vi "Show Error Details.vi"(8 "error in (no error)":errorcluster, 10 "Error Info":T1 {"Time Stamp" format="%<%x %.3X>T"}, 11 "Error Manager in":refnum<class "Local Error Manager.lvclass">) -> (0 "error out":errorcluster, 3 "Error Manager out":refnum<class "Local Error Manager.lvclass">)   [LabVIEW 2026, in "TALOS.lvlib" / "Error Manager.lvlib" / "Local Error Manager.lvclass"]
uses:
  Local Error Manager.lvclass
  C:/LabVIEW Code/TALOS/talos/Father of all uServices/Father of all uServices/Father of all uServices.lvclass
  Error Info.ctl
  Local Error Manager.lvclass/Local Error Manager.ctl
  Ancestor/Ancestor/Ancestor.lvclass/Ancestor.ctl
  <vilib>/AdvancedString/Delimited String to 1D String Array (string).vi
  Support VIs/Generate Error.vi
  FGV/Error Memory/Get Error Description.vi
  Support VIs/Get PC name.vi
  Ancestor/Ancestor/Read ID.vi
  Support VIs/Get Class Name.vi
  FGV/Error Memory/Error Memory Core.vi
  Support VIs/Circus Root Path.vi
  FGV/Error Memory/Error Crt Lvl checker.vi
  FGV/Error Memory/Error Memory Core.vi/40c8088d-b597-4017-91af-faa98e00292e.vi
  FGV/Error Memory/Error Memory Core.vi/d4a3ab98-063c-4e44-b43d-fbdcfe6c2be2.vi
  Support VIs/Global Memory.vi
  <vilib>/Utility/LVClass/Get LV Class Name.vi
  Support VIs/Is in Packed Library.vi
  Support VIs/TALOS Root path.vi
  Support VIs/Read CSV worksheet.vi
  Support VIs/Global Constants.vi
  <vilib>/Utility/error.llb/General Error Handler.vi
  Support VIs/Error Log.vi
  Ancestor/Ancestor/Ancestor.lvclass
  <vilib>/Comparison/Equal/Equal Functor/Equal Functor.lvclass
  Father of all uServices/Father of all uServices/Father of all uServices.lvclass
  TALOS.lvlib
  Error Manager.lvclass
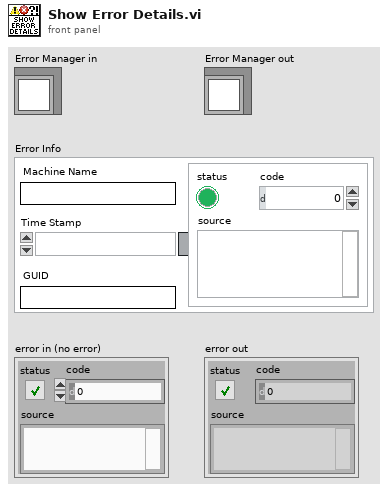
[diagram p1: front panel]
types:
  T1 = typedef "TALOS.lvlib/Error Manager.lvlib/Error Manager.lvclass/Error Info.ctl" = cluster{"error out":errorcluster, "Time Stamp":timestamp, "Machine Name":string, "GUID":string}
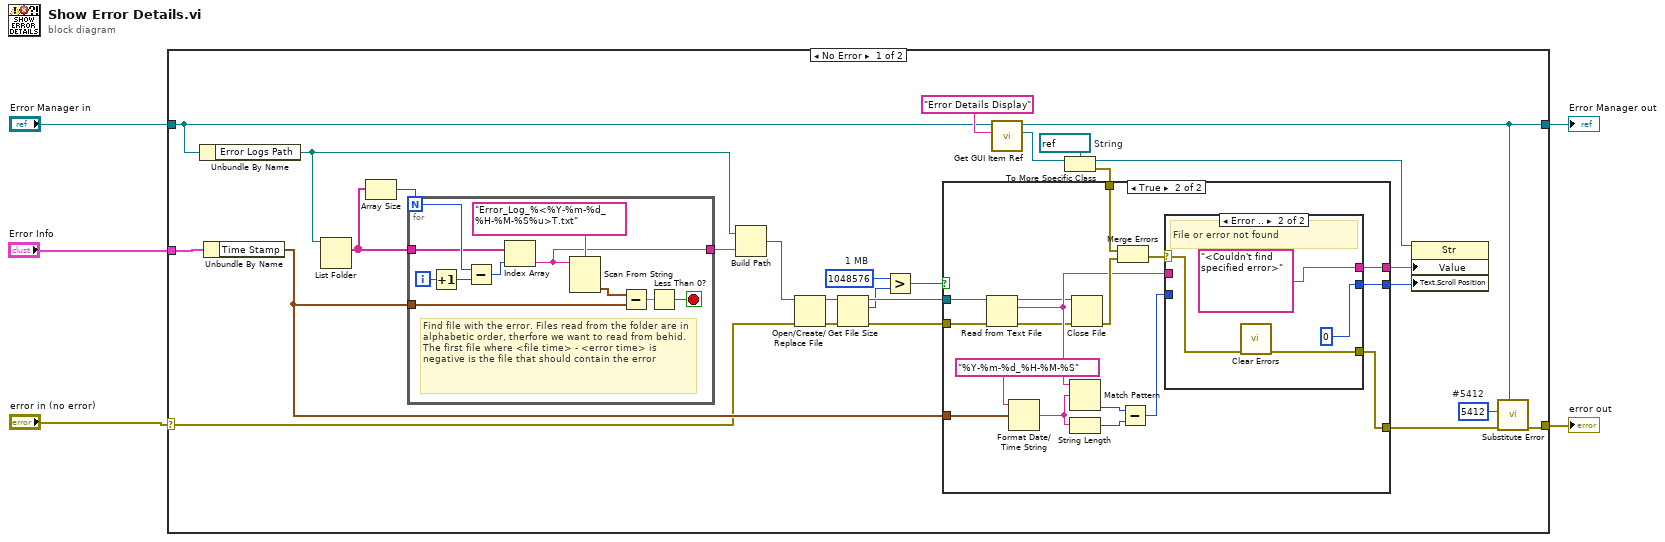
[diagram p0: block diagram]
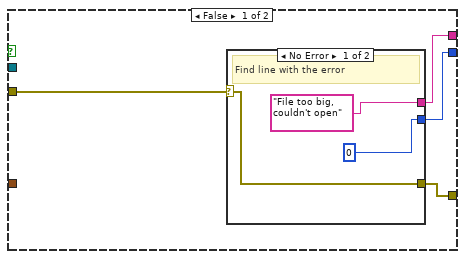
[diagram p2: hidden frame]
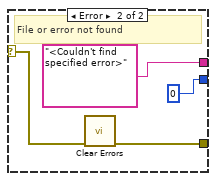
[diagram p3: hidden frame]
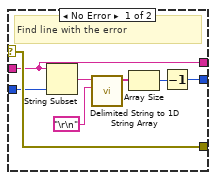
[diagram p4: hidden frame]
diagram:
  n1 = case shown="No Error" "error in (no error)" {
    selector: "error in (no error)" -> [w25 w84]
    tunnel: [w7 w84] -> w5
    tunnel: [w6 w85] -> w4
    tunnel: "Error Manager in" -> [w23 w85]
    tunnel: "Error Info" -> [w17 _]
    frame No Error {
      w9 = 5412  # #5412
      w11 = i64 1048576  # 1 MB
      w28 = refnum<vi> refnum  # String
      n2 = Unbundle By Name(w23) -> ("Error Logs Path"=w18:path)
      n3 = Unbundle By Name(w17) -> ("Time Stamp"=w29:timestamp)
      n4 = List Folder(path=w18) -> (filenames=w20:string[])  [unwired: 3 in, 3 out]
      n5 = Array Size(array=w20) -> (size(s)=w19:i32)
      n6 = for {
        N: w19 -> [w82]
        tunnel: w20 -> [w80]
        tunnel: w29 -> [w76]
        tunnel: [w73] -> w21
        i -> [w83]
        stop <- w74 stop-if-true
        # "Find file with the error. Files read from the folder are in alphabetic order, therfore we want to read from behid. The first file where <file time> - <error time> is negative is the file that should contain the error"
        n7 = Increment(x=w83) -> (x+1=w81:i32)
        n8 = Subtract(x=w82, y=w81) -> (x-y=w79:i32)
        n9 = Index Array(array=w80, index=w79) -> (element=w73:string)
        n10 = Scan From String(format string="Error_Log_%<%Y-%m-%d_%H-%M-%S%u>T.txt", input string=w73) -> (output 1=w77:timestamp)  [unwired: 3 in, 3 out]
        n11 = Subtract(x=w77, y=w76) -> (x-y=w75:dbl)
        n12 = Less Than 0?(x=w75) -> (x < 0?=w74:bool)
      }
      n13 = Build Path(base path=w18, name or relative path=w21) -> (appended path=w22:path)
      n14 = Open/Create/Replace File(file path (use dialog)=w22, error in=w25) -> (refnum out=w15:refnum<file>, error out=w16:errorcluster)  [unwired: 4 in, 1 out]
      n15 = Get File Size(file=w15, error in=w16) -> (refnum out=w14:refnum<file>, size (in bytes)=w12:i64, 0:w13:errorcluster)
      n16 = Greater?(x=w11, y=w12) -> (0:w10:bool)
      n17 = call "Get GUI Item Ref.vi"("FP Item Name"="Error Details Display", "uService Template in"=w23) -> ("Ctl Refnum"=w26:refnum<vi>, "uService Template out"=w6:refnum<class "Local Error Manager.lvclass">)  [unwired: 7 in, 1 out]
      n18 = To More Specific Class(target class=w28, reference=w26) -> (specific class reference=w27:refnum<vi>, error out=w31:errorcluster)  [unwired: 1 in]
      n19 = case shown="True" w10 {
        tunnel: [w35 w60] -> w8
        tunnel: [w34 w59] -> w32
        tunnel: w31 -> [_ w56]
        tunnel: [w33 w54] -> w30
        tunnel: w29 -> [_ w48]
        tunnel: w14 -> [_ w45]
        tunnel: w13 -> [w36 w44]
        frame False {
          n20 = case shown="No Error" w36 {
            selector: w36 -> [w39 w41]
            tunnel: [0 0] -> w33
            tunnel: ["File too big, couldn't open" "<Couldn't find specified error>"] -> w34
            tunnel: [w39 w40] -> w35
            frame No Error {
              # "Find line with the error"
            }
            frame Error {
              # "File or error not found"
              n21 = call <vilib>:"Clear Errors.vi"("error in (no error)"=w41) -> ("error out"=w40:errorcluster)  [unwired: 5 in, 1 out]
            }
          }
        }
        frame True {
          n22 = Read from Text File(file (use dialog)=w45, error in=w44) -> (refnum out=w47:refnum<file>, text=w53:string, error out=w46:errorcluster)  [unwired: 2 in, 1 out]
          n23 = Format Date/Time String(time format string (%c)="%Y-%m-%d_%H-%M-%S", seconds (now)=w48) -> (date/time string=w51:string)  [unwired: 1 in]
          n24 = Match Pattern(string=w53, regular expression=w51) -> (offset past match=w52:i32)  [unwired: 1 in, 3 out]
          n25 = String Length(string=w51) -> (length=w50:i32)
          n26 = Close File(refnum=w47, error in=w46) -> (error out=w57:errorcluster)  [unwired: 1 out]
          n27 = Merge Errors(w56, w57) -> (w58:errorcluster)
          n28 = Subtract(x=w52, y=w50) -> (x-y=w55:i32)
          n29 = case shown="Error .." w58 {
            selector: w58 -> [w68 w70]
            tunnel: w53 -> [w61 _]
            tunnel: [w63 0] -> w54
            tunnel: w55 -> [w62 _]
            tunnel: [w61 "<Couldn't find specified error>"] -> w59
            tunnel: [w68 w69] -> w60
            frame No Error {
              # "Find line with the error"
              n30 = String Subset(string=w61, length (rest)=w62) -> (substring=w64:string)  [unwired: 1 in]
              n31 = call-poly <vilib>:"Delimited String to 1D String Array.vi"("delimiter"="\r\n", "delimited string"=w64) -> ("string array"=w66:string[])  [unwired: 9 in]
              n32 = Array Size(array=w66) -> (size(s)=w65:i32)
              n33 = Decrement(x=w65) -> (x-1=w63:i32)
            }
            frame Error {
              # "File or error not found"
              n34 = call <vilib>:"Clear Errors.vi"("error in (no error)"=w70) -> ("error out"=w69:errorcluster)  [unwired: 5 in, 1 out]
            }
          }
        }
      }
      n35 = property class="Str"(reference=w27, "Value"=w32, "Text.Scroll Position"=w30) -> ()  [unwired: 1 in, 2 out]
      n36 = call "Substitute Error.vi"("LabVIEW Object"=w6, "error in (no error)"=w8, "Error Code"=w9) -> ("error out"=w7:errorcluster)  [unwired: 8 in]
    }
    frame Error {
    }
  }
  "error out" <- w5
  "Error Manager out" <- w4
